vi "_toml_example.vi"() -> ()   [LabVIEW 2017]
uses:
  toml_value_operation.ctl
panel:
  out "error out":errorcluster
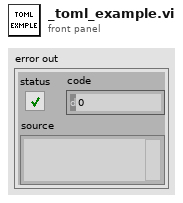
[diagram p1: front panel]
types:
  T1 = typedef "toml_value_operation.ctl" = enum8{"read", "write", "delete"}
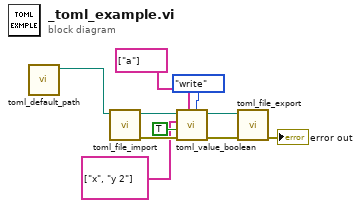
[diagram p0: block diagram]
diagram:
  n1 = call "toml_default_path.vi"() -> ("app.toml"=w10:path)  [unwired: 9 in, 2 out]
  n2 = call "toml_file_import.vi"("path in"=w10) -> ("error out"=w9:errorcluster, "path out"=w7:path)  [unwired: 9 in]
  n3 = call "toml_value_boolean.vi"("operation"=toml_value_operation."write", "section"=string[] ["a"], "error in (no error)"=w9, "value in"=TRUE, "key"=string[] ["x", "y 2"], "path in"=w7) -> ("error out"=w8:errorcluster, "path out"=w6:path)  [unwired: 2 in, 2 out]
  n4 = call "toml_file_export.vi"("error in (no error)"=w8, "path in"=w6) -> ("error out"=→"error out":errorcluster)  [unwired: 8 in, 1 out]
